vi "TrapRaster2Offset.vi"() -> (3 "OffAX":dbl[](array[numeric]) format="%_6g")   [LabVIEW 2014]
uses:
  <vilib>/gmath/NI_Gmath.lvlib
panel:
  out "OffBX":dbl[](array[numeric]) format="%_6g"
  out "OffTD":dbl[](array[numeric])
  in  "dTD":dbl=0.1
  in  "Path":path
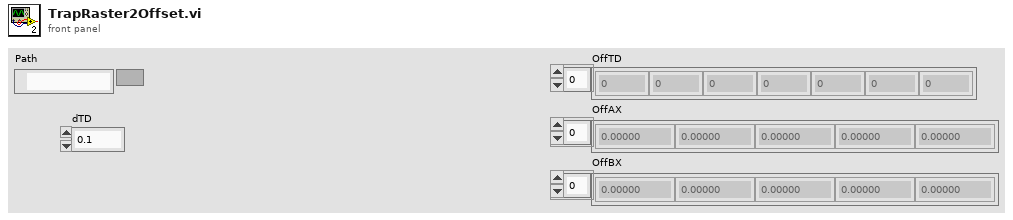
[diagram p1: front panel]
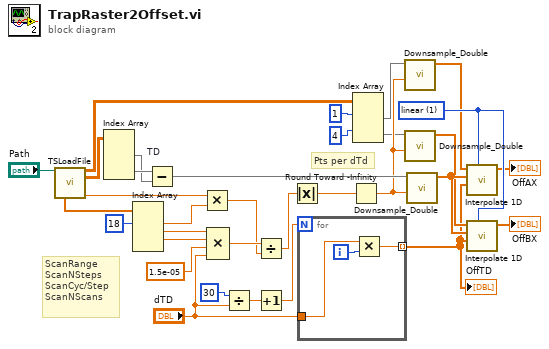
[diagram p0: block diagram]
diagram:
  w15 = 1 items=["nearest", "linear", "spline", "cubic Hermite", "Lagrange"] ("method")
  # "Pts per dTd"
  # "ScanRange\nScanNSteps\nScanCyc/Step\nScanNScans"
  n1 = call "TSLoadFile.vi"("Path"="Path") -> ("Trap"=w21:dbl[][], "TPos"=w26:dbl[][], "Hdr"=w32:dbl[], "Fs"=w1:dbl)  [unwired: 8 in, 3 out]
  n2 = Index Array(array=w26) -> (element #1=w24:dbl[], element #2=w25:dbl[])  [unwired: 4 in]
  n3 = Index Array(array=w32, index #1=18 ("index")) -> (element #1=w2:dbl, element #2=w3:dbl, element #3=w5:dbl)  [unwired: 3 in, 1 out]
  n4 = Subtract "TD"(x=w25, y=w24) -> (x-y=w23:dbl[])
  n5 = Multiply(x=w1, y=w2) -> (x*y=w28:dbl)
  n6 = Compound Arithmetic op=MULTIPLY(w3, w5, 1.5e-05 ("value"), "dTD") -> (w29:dbl)
  n7 = Divide(x=30, y="dTD") -> (x/y=w11:dbl)
  n8 = Divide(x=w29, y=w28) -> (x/y=w27:dbl)
  n9 = Increment(x=w11) -> (x+1=w10:dbl)
  n10 = Absolute Value(x=w27) -> (abs(x)=w4:dbl)
  n11 = for {
    N: w10 -> [_]
    tunnel: "dTD" -> [w35]
    tunnel: [w34] -> w6 mode=indexing
    i -> [w36]
    n12 = Multiply(x=w35, y=w36) -> (x*y=w34:dbl)
  }
  "OffTD" <- w6
  n13 = Round Toward -Infinity(1:w4) -> (0:w22:dbl)
  n14 = Index Array(array=w21, index (row) #1=1, index (row) #2=4) -> (element #1=w18:dbl[], element #2=w17:dbl[])  [unwired: 2 in]
  n15 = call "Downsample_Double.vi"("Ave N"=w22, "Array In"=w18) -> ("Array Out"=w13:dbl[])  [unwired: 9 in]
  n16 = call "Downsample_Double.vi"("Ave N"=w22, "Array In"=w17) -> ("Array Out"=w14:dbl[])  [unwired: 9 in]
  n17 = call "Downsample_Double.vi"("Ave N"=w22, "Array In"=w23) -> ("Array Out"=w16:dbl[])  [unwired: 9 in]
  n18 = call <vilib>:"Interpolate 1D.vi"("method"=w15, "xi"=w6, "X"=w16, "Y"=w13) -> ("yi"=→"OffAX":dbl[])  [unwired: 5 in, 2 out]
  n19 = call <vilib>:"Interpolate 1D.vi"("method"=w15, "xi"=w6, "X"=w16, "Y"=w14) -> ("yi"=→"OffBX":dbl[])  [unwired: 5 in, 2 out]
